vi "Waveform and XY Plots.vi"() -> (1 "xy plot":picture, 2 "waveform plot":picture)   [LabVIEW 2012]
doc: "Uses the Plot Waveform VI and Plot XY VI to draw a waveform and XY graph in a picture indicator.\n\nNote: You must have the LabVIEW Full or Professional Development Systems to run this example."
panel:
  # "This simple example shows how the Plot Waveform and Plot XY VIs can be used.\nThe only input to the VIs is the data which is automatically\nscaled and plotted in the picture control."
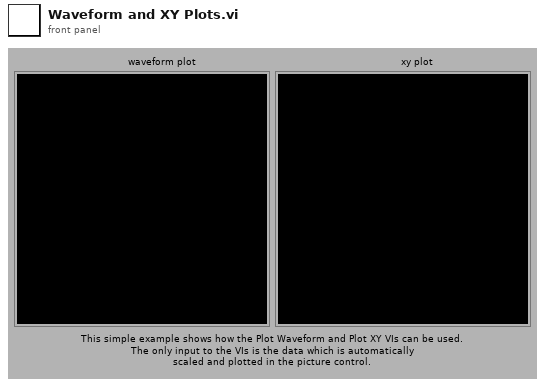
[diagram p1: front panel]
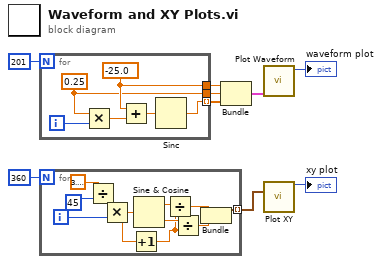
[diagram p0: block diagram]
diagram:
  n1 = for {
    N: 201 -> [_]
    tunnel: [w13] -> w7 mode=indexing
    tunnel: [w12] -> w6
    tunnel: [w10] -> w5
    i -> [w15]
    w12 = -25.0
    w10 = 0.25
    n2 = Multiply(x=w10, y=w15) -> (x*y=w14:dbl)
    n3 = Add(x=w12, y=w14) -> (x+y=w11:dbl)
    n4 = Sinc(1:w11) -> (0:w13:dbl)
  }
  n5 = for {
    N: 360 -> [_]
    tunnel: [w25] -> w1 mode=indexing
    i -> [w16]
    n6 = Divide(x=3.141592653589793, y=45) -> (x/y=w26:dbl)
    n7 = Multiply(x=w26, y=w16) -> (x*y=w18:dbl)
    n8 = Increment(x=w18) -> (x+1=w17:dbl)
    n9 = Sine & Cosine(0:w18) -> (1:w22:dbl, 2:w20:dbl)
    n10 = Divide(x=w22, y=w17) -> (x/y=w21:dbl)
    n11 = Divide(x=w20, y=w17) -> (x/y=w19:dbl)
    n12 = Bundle(w21, w19) -> (w25:cluster{dbl, dbl})  [unwired: 1 out]
  }
  n13 = Bundle(w6, w5, w7) -> (w4:cluster{dbl, dbl, dbl[]})  [unwired: 1 out]
  n14 = call <vilib>:"Plot Waveform.vi"("waveform data"=w4) -> ("new picture"=→"waveform plot":picture)  [unwired: 8 in, 2 out]
  n15 = call <vilib>:"Plot XY.vi"("data"=w1) -> ("new picture"=→"xy plot":picture)  [unwired: 5 in, 9 out]
